vi "Get Active Controller.vi"(8 "error in (no error)":errorcluster, 11 "Vessel in":refnum<class "Vessel.lvclass">) -> (0 "error out":errorcluster, 2 "Controller Out":refnum<class "Controller.lvclass">, 3 "Vessel out":refnum<class "Vessel.lvclass">)   [LabVIEW 2014, in "Vessel.lvclass"]
uses:
  Vessel.lvclass
  Controller/Controller.lvclass
  Vessel.lvclass/Vessel.ctl
  Supervisor/Supervisor.lvclass
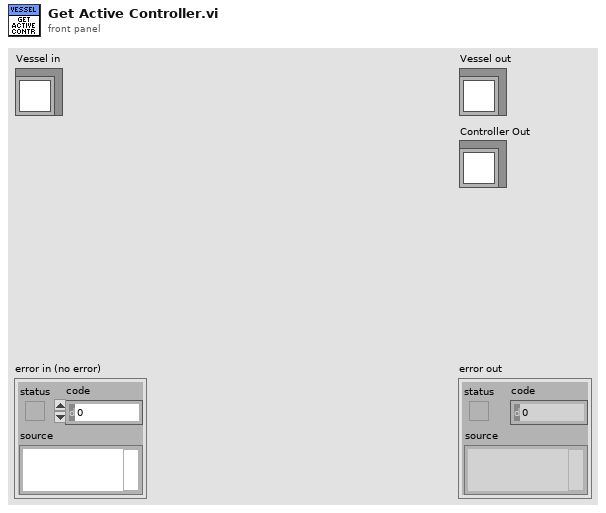
[diagram p1: front panel]
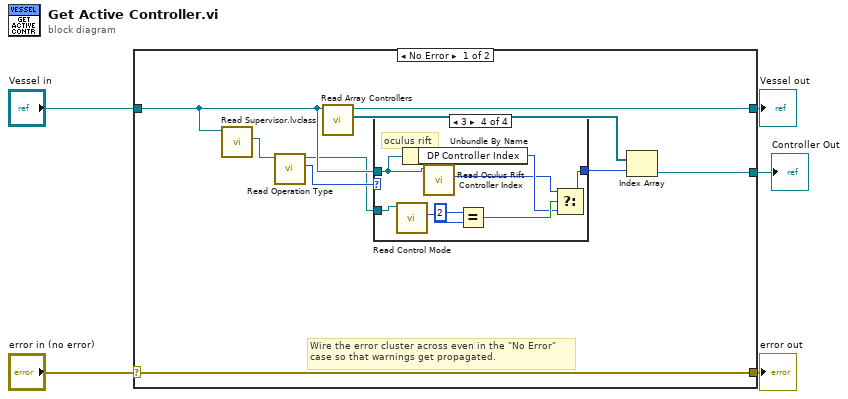
[diagram p0: block diagram]
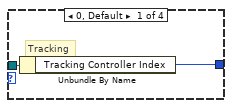
[diagram p2: hidden frame]
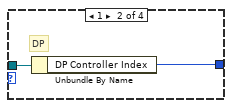
[diagram p3: hidden frame]
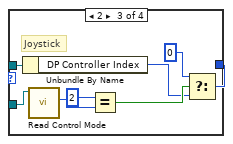
[diagram p4: hidden frame]
diagram:
  n1 = case shown="No Error" "error in (no error)" {
    selector: "error in (no error)" -> [w14 w36]
    tunnel: [w14 w36] -> w4
    tunnel: [w9 w35] -> w2
    tunnel: "Vessel in" -> [w8 w35]
    tunnel: [w10 _] -> w1
    frame No Error {
      # "Wire the error cluster across even in the \"No Error\"\ncase so that warnings get propagated."
      n2 = call "Read Supervisor.lvclass.vi"("Vessel in"=w8) -> ("Supervisor.lvclass"=w13:refnum<class "Supervisor.lvclass">)  [unwired: 8 in, 2 out]
      n3 = call-dynamic "Read Operation Type.vi"("Supervisor in"=w13) -> ("Operation Type"=w12:u16, "Supervisor out"=w6:refnum<class "Supervisor.lvclass">)  [unwired: 8 in, 1 out]
      n4 = call "Read Array Controllers.vi"("Vessel in"=w8) -> ("Array Controllers"=w7:refnum<class "Controller.lvclass">[], "Vessel out"=w9:refnum<class "Vessel.lvclass">)  [unwired: 8 in, 1 out]
      n5 = case shown="3" w12 {
        tunnel: w8 -> [w16 w18 w26 w29]
        tunnel: [w15 w17 w20 w31] -> w11
        tunnel: w6 -> [_ _ w25 w30]
        frame 0, Default {
          # "Tracking"
          n6 = Unbundle By Name(w16) -> ("Tracking Controller Index"=w15:i32)
        }
        frame 1 {
          # "DP"
          n7 = Unbundle By Name(w18) -> ("DP Controller Index"=w17:i32)
        }
        frame 2 {
          # "Joystick"
          n8 = Unbundle By Name(w26) -> ("DP Controller Index"=w21:i32)
          n9 = call-dynamic "Read Control Mode.vi"("Supervisor in"=w25) -> ("Control Mode"=w24:u16)  [unwired: 8 in, 2 out]
          n10 = Equal?(x=u16 2, y=w24) -> (x = y?=w22:bool)
          n11 = Select(t=0, s=w22, f=w21) -> (s? t:f=w20:i32)
        }
        frame 3 {
          # "oculus rift"
          n12 = call-dynamic "Read Control Mode.vi"("Supervisor in"=w30) -> ("Control Mode"=w34:u16)  [unwired: 8 in, 2 out]
          n13 = Unbundle By Name(w29) -> ("DP Controller Index"=w28:i32)
          n14 = call-dynamic "Read Oculus Rift Controller Index.vi"("Vessel in"=w29) -> ("Oculus Rift Controller Index"=w27:i32)  [unwired: 8 in, 2 out]
          n15 = Equal?(x=u16 2, y=w34) -> (x = y?=w32:bool)
          n16 = Select(t=w27, s=w32, f=w28) -> (s? t:f=w31:i32)
        }
      }
      n17 = Index Array(array=w7, index=w11) -> (element=w10:refnum<class "Controller.lvclass">)
    }
    frame Error {
    }
  }
  "error out" <- w4
  "Vessel out" <- w2
  "Controller Out" <- w1
